vi "ClassPanel.vi"(8 "error in (no error)":errorcluster caption="entrée d'erreur (pas d'erreur)", 11 "SR530.lvclass":refnum<class "SR530.lvclass">) -> (0 "error out":errorcluster caption="sortie d'erreur", 3 "SR530.lvclass Out":refnum<class "SR530.lvclass">)   [LabVIEW 2019, in "SR530.lvclass"]
uses:
  SR530.lvclass
  C:/Programmes Labview/LabscanV1A/DevicesClass/BaseDevice/BaseDevice.lvclass
  <userlib>/SR530/Inputs.ctl
  <userlib>/SR530/ReadParam.ctl
  <userlib>/SR530/SetParam.ctl
  BaseDevice/ClassQueueMess.ctl
  BaseDevice/Accessor/GetClassEvent.vi
panel:
  in  "Read:":T1 items=["Channel 1", "X Output", "Channel 2", "Y Output", "X1", "X2", "X3", "X4", "X5", "X6", "Ch1 and Ch2", "X and Y", "X,Y,Ch1,Ch2"]
  in  "MainProgQ":refnum<queue>
  in  "MainProgQEvent":refnum<user-event>
  in  "Pre Time":u16(ring)=1 items=["1 ms"=1, "3 ms"=2, "10 ms"=3, "30 ms"=4, "100 ms"=5, "300 ms"=6, "1 s"=7, "3 s"=8, "10 s"=9, "30 s"=10, "100 s"=11]
  in  "Sensitivity":u16(ring)=1 items=["10 nV"=1, "20 nV"=2, "50 nV"=3, "100 nV"=4, "200 nV"=5, "500 nV"=6, "1 µV"=7, "2 µV"=8, "5 µV"=9, "10 µV"=10, "20 µV"=11, "50 µV"=12, "100µV"=13, "200 µV"=14, "500µV"=15, "1 mV"=16, "2 mV"=17, "5 mV"=18, "10 mV"=19, "20 mV"=20, "50 mV"=21, "100 mV"=22, "200mV"=23, "500 mV"=24]
  in  "Acq":bool
  out "Phase":dbl=1000.0 caption="Phase (°)" min=0.0 step=0.1 format="%#_5f"
  out "MAG":dbl=1000.0 caption="MAG (V)" min=0.0 step=0.1 format="%^#_6e"
  out "UNLCK":bool caption="SpexMov"
  out "X":dbl=1000.0 caption="X (V)" min=0.0 step=0.1 format="%^#_6e"
  in  "Stop":bool
  out "Init Program":bool
  out "OVLD":bool caption="SpexMov"
  in  "Update":bool caption="stopSpectro"
  out "Y":dbl=1000.0 caption="Y (V)" min=0.0 step=0.1 format="%^#_6e"
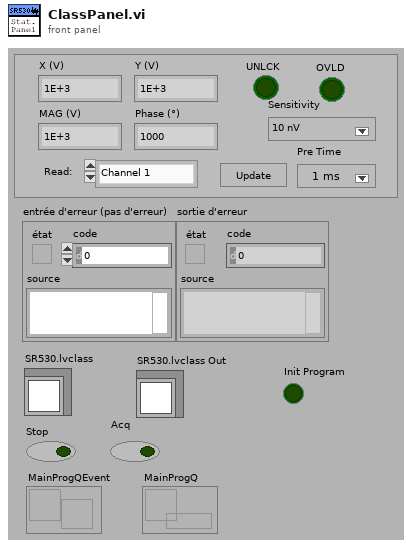
[diagram p1: front panel]
types:
  T1 = typedef "Inputs.ctl" = u16
  T2 = typedef "ReadParam.ctl" = enum16{"BandPass Filter", "Dynamic Reserve", "Expand", "Frequency", "Ref Trig", "Ch Settings", "Gain", "Notch Filter", "Time Constant", "All", "End"}
  T3 = typedef "SetParam.ctl" = enum16{"BandPass Filter", "Dynamic Reserve", "Expand", "Ref Trig", "Ch Settings", "Gain", "Notch Filter", "Pre Time Constant", "Post Time Constant"}
  T4 = cluster{"Channel":u16, "Outputs":dbl[], "Status Byte":bool[]}
  T5 = enum16{"Enable", "Disable", "DisAndGrayed", "ReinitToDefVal", "EnumElementsArr"}
  T6 = enum8{"Enabled", "Disabled", "Disabled and Grayed Out"}
  T7 = cluster{"BandFilter":bool, "LineFilter1x":bool, "LineFilter2x":bool, "Expand Ch1":bool, "Expand Ch2":bool, "Sensitivity":u16, "Pre Time":u16, "Post Time":u16, "Dynamic Res.":u16, "Reference Trigger":u16, "Channels Settings":u16, "Frequency":dbl}
  T8 = typedef "ClassQueueMess.ctl" = u16
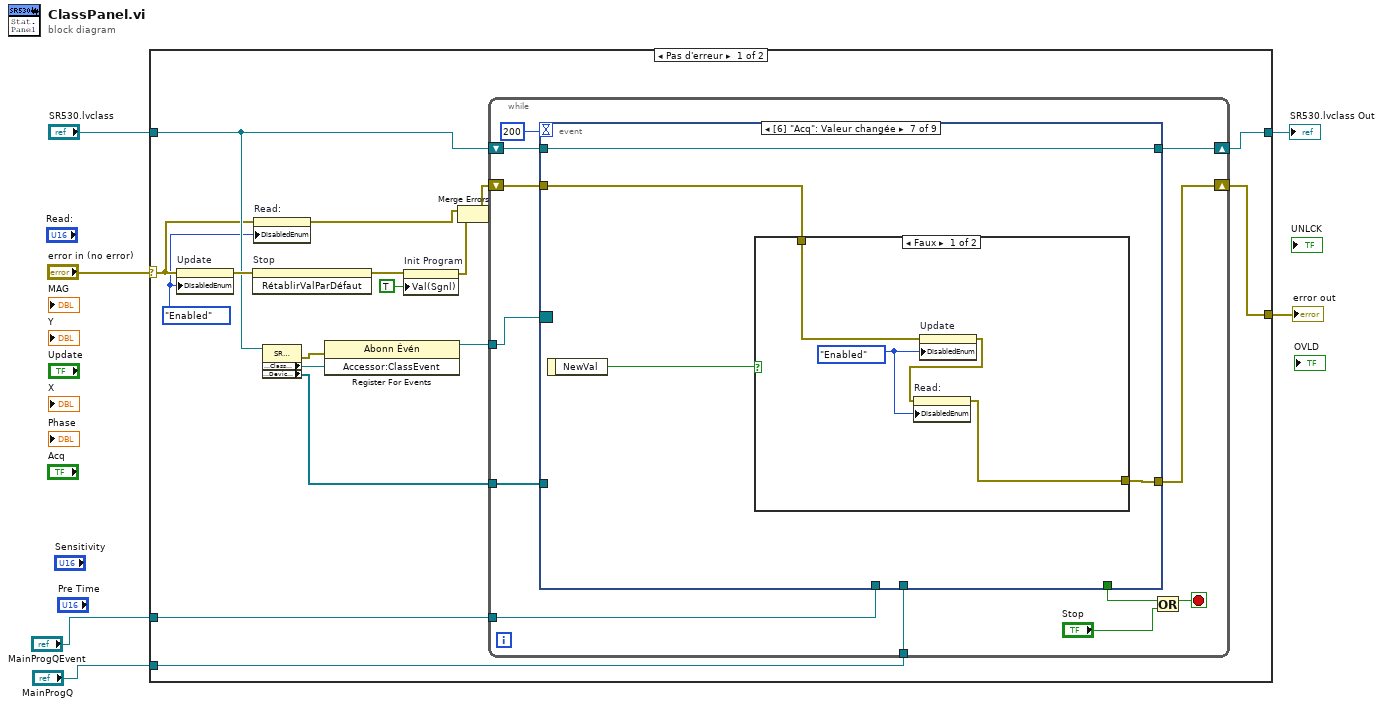
[diagram p0: block diagram]
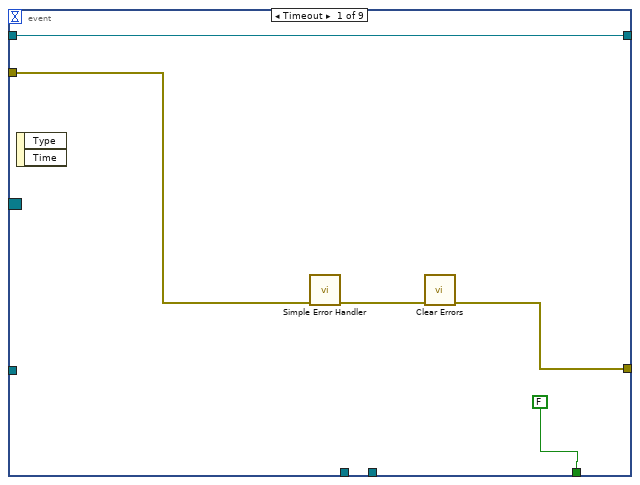
[diagram p2: hidden frame]
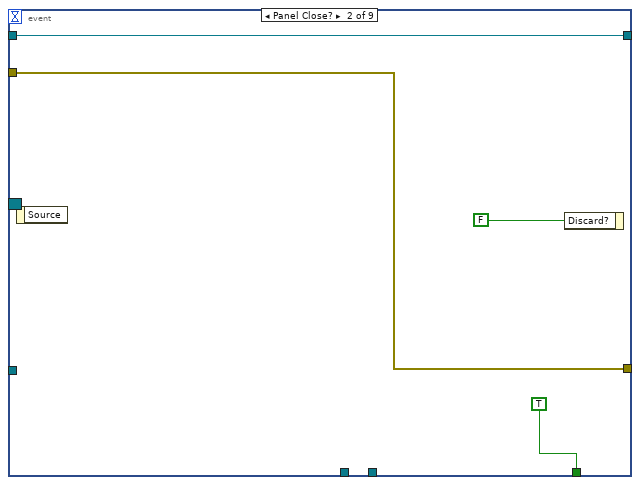
[diagram p3: hidden frame]
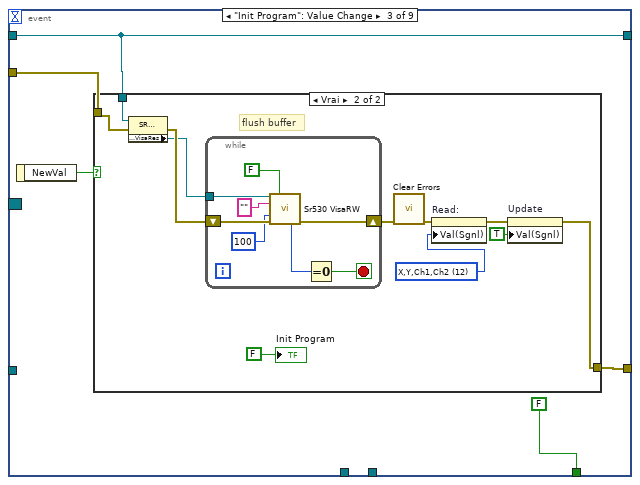
[diagram p4: hidden frame]
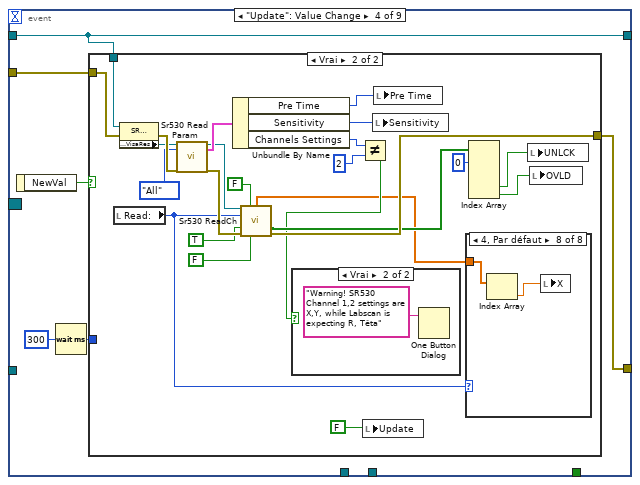
[diagram p6: hidden frame]
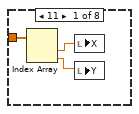
[diagram p8: hidden frame]
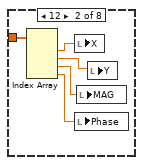
[diagram p9: hidden frame]
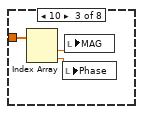
[diagram p10: hidden frame]
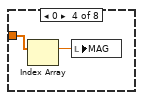
[diagram p11: hidden frame]
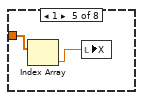
[diagram p12: hidden frame]
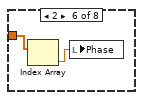
[diagram p13: hidden frame]
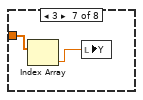
[diagram p14: hidden frame]
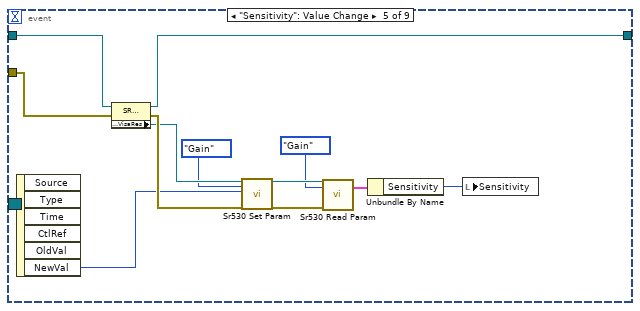
[diagram p16: hidden frame]
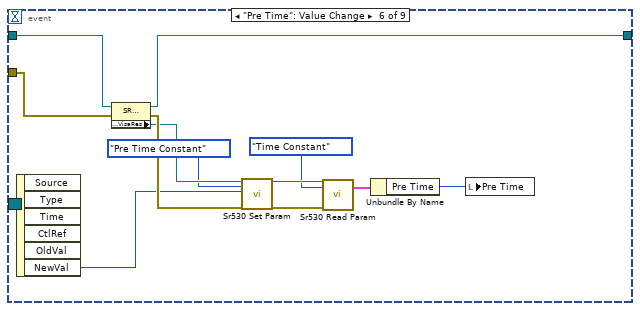
[diagram p17: hidden frame]
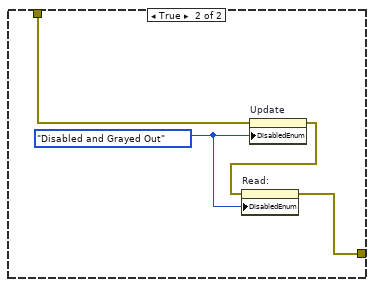
[diagram p18: hidden frame]
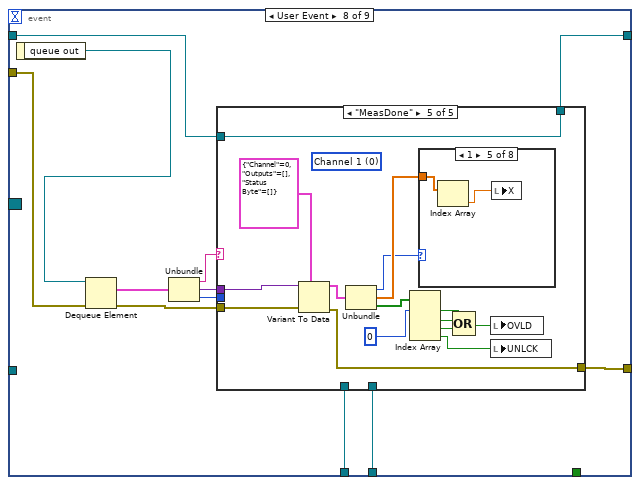
[diagram p19: hidden frame]
diagram:
  n1 = case shown="Pas d'erreur" "error in (no error)" {
    selector: "error in (no error)" -> [w10 w358]
    tunnel: [w14 w358] -> w5
    tunnel: "SR530.lvclass" -> [w15 w357]
    tunnel: [w22 w357] -> w3
    tunnel: "MainProgQEvent" -> [w13 _]
    tunnel: "MainProgQ" -> [w12 _]
    frame No Error {
      w7 = T6."Enabled" ("Désactivé")
      n2 = property on="Update" class="Bool (strict)"(error in=w10, "DisabledEnum"=w7) -> (error out=w18:errorcluster)  [unwired: 1 in, 1 out]
      n3 = invoke on="Stop" class="Bool (strict)" method="RétablirValParDéfaut"(error in=w18) -> (error out=w21:errorcluster)  [unwired: 2 in, 2 out]
      n4 = property on="Read:" class="MDér (strict)"(error in=w10, "DisabledEnum"=w7) -> (error out=w8:errorcluster)  [unwired: 1 in, 1 out]
      n5 = property class="SR530.lvclass"(reference=w15) -> (error out=w19:errorcluster, "Accessor:ClassEvent"=w20:refnum<user-event>, "Accessor:DeviceCtrl"=w11:refnum<vi>[])  [unwired: 1 in, 1 out]
      n6 = register-events(error in=w19, w20) -> (reference out=w17:refnum<event-registration>)  [unwired: 1 in, 1 out]
      n7 = property on="Init Program" class="Bool (strict)"(error in=w21, "Val(Sgnl)"=TRUE ("Valeur (Signalisation)")) -> (error out=w16:errorcluster)  [unwired: 1 in, 1 out]
      n8 = Merge Errors(w8, w16) -> (w9:errorcluster)
      n9 = while {
        shift-right: [w33] -> w14
        shift-left: w9 -> [w34]
        shift-right: [w30] -> w22
        shift-left: w15 -> [w32]
        tunnel: w17 -> [w27]
        tunnel: w13 -> [w26]
        tunnel: w12 -> [w25]
        tunnel: w11 -> [w24]
        stop <- w29 stop-if-true
        n10 = event shown="[6] \"Acq\": Valeur changée" {
          selector: w27 -> [_ _ _ _ _ _ _ _ _]
          dyn-events: _ -> [_ _ _ _ _ _ _ _ _]
          timeout: 200 -> [_ _ _ _ _ _ _ _ _]
          tunnel: w34 -> [w38 w42 w48 w70 w132 w144 w150 w168 w233]
          tunnel: [w36 w42 w47 w74 _ _ w148 w161 w234] -> w33
          tunnel: w32 -> [w39 w41 w45 w71 w133 w145 w147 w164 w242]
          tunnel: [FALSE TRUE FALSE _ _ _ _ _ _] -> w31
          tunnel: [w39 w41 w45 w71 w131 w143 w147 w163 w236] -> w30
          tunnel: w26 -> [_ _ _ _ _ _ _ w160 _]
          tunnel: w25 -> [_ _ _ _ _ _ _ w159 _]
          tunnel: w24 -> [_ _ _ _ _ _ _ _ w239]
          event Timeout {
            n11 = event-data() -> ()  [unwired: 1 in, 2 out]
            n12 = call <vilib>:"Simple Error Handler.vi"("error in (no error)"=w38) -> ("error out"=w37:errorcluster)  [unwired: 4 in, 4 out]
            n13 = call <vilib>:"Clear Errors.vi"("error in (no error)"=w37) -> ("error out"=w36:errorcluster)  [unwired: 5 in, 1 out]
          }
          event Panel Close? {
            n14 = event-data() -> ()  [unwired: 1 in, 1 out]
            n15 = event-data("Discard?"=FALSE ("Rejeter ?")) -> ()  [unwired: 1 in, 1 out]
          }
          event "Init Program": Value Change {
            n16 = event-data() -> ("NewVal"=w49:bool)  [unwired: 1 in]
            n17 = case shown="Vrai" w49 {
              tunnel: w48 -> [w50 w57]
              tunnel: [w50 w59] -> w47
              tunnel: w45 -> [_ w56]
              frame False {
              }
              frame True {
                w51 = T1 12 items=["Channel 1", "X Output", "Channel 2", "Y Output", "X1", "X2", "X3", "X4", "X5", "X6", "Ch1 and Ch2", "X and Y", "X,Y,Ch1,Ch2"] ("Read:")
                # "flush buffer"
                n18 = property class="SR530.lvclass"(reference=w56, error in=w57) -> (error out=w55:errorcluster, "Accessor:VisaRes"=w54:refnum<visa-resource-name>)  [unwired: 1 out]
                n19 = while {
                  tunnel: w54 -> [w68]
                  shift-right: [w64] -> w58
                  shift-left: w55 -> [w69]
                  stop <- w62 stop-if-true
                  n20 = call <userlib>:"Sr530 VisaRW.vi"("VISA Rsrc"=w68, "2Lecture?"=FALSE, "ChaineCom"="", "Nbcaract"=u32 100, "error in (no error)"=w69) -> ("Count out"=w63:u32, "error out"=w64:errorcluster)  [unwired: 5 in, 4 out]
                  n21 = Equal To 0?(x=w63) -> (x = 0?=w62:bool)
                }
                n22 = call <vilib>:"Clear Errors.vi"("error in (no error)"=w58) -> ("error out"=w52:errorcluster)  [unwired: 5 in, 1 out]
                n23 = property on="Read:" class="MDér (strict)"(error in=w52, "Val(Sgnl)"=w51) -> (error out=w53:errorcluster)  [unwired: 1 in, 1 out]
                n24 = property on="Update" class="Bool (strict)"(error in=w53, "Val(Sgnl)"=TRUE ("Valeur (Signalisation)")) -> (error out=w59:errorcluster)  [unwired: 1 in, 1 out]
                "Init Program" <- FALSE
              }
            }
          }
          event "Update": Value Change {
            n25 = event-data() -> ("NewVal"=w75:bool)  [unwired: 1 in]
            n26 = Wait (ms)(milliseconds to wait=u32 300 ("attente (ms)")) -> (millisecond timer value=w72:u32)
            n27 = case shown="Vrai" w75 {
              tunnel: w70 -> [w76 w93]
              tunnel: [w76 w87] -> w74
              tunnel: w72 -> [_ _]
              tunnel: w71 -> [_ w96]
              frame False {
              }
              frame True {
                n28 = local read "Read:"() -> (w78:T1)
                n29 = property class="SR530.lvclass"(reference=w96, error in=w93) -> (error out=w95:errorcluster, "Accessor:VisaRes"=w94:refnum<visa-resource-name>)  [unwired: 1 out]
                n30 = call <userlib>:"Sr530 Read Param.vi"("Ressource VISA"=w94, "Param"=ReadParam."All", "error in (no error)"=w95) -> ("Ressource VISA Out"=w91:refnum<visa-resource-name>, "LockInPar"=w100:T7, "error out"=w92:errorcluster)  [unwired: 13 in, 1 out]
                n31 = Unbundle By Name(w100) -> ("Pre Time"=w80:u16, "Sensitivity"=w99:u16, "Channels Settings"=w83:u16)
                n32 = call <userlib>:"Sr530 ReadCh.vi"("VISA Rsrc"=w91, "Autoscale"=FALSE, "Channel"=w78, "Check Status"=TRUE, "error in (no error)"=w92, "Ask Correction"=FALSE) -> ("Outputs"=w77:dbl[], "Status Byte"=w86:bool[], "error out"=w87:errorcluster)  [unwired: 2 in, 5 out]
                n33 = Not Equal?(x=w83, y=u16 2 ("Channels Settings")) -> (x != y?=w81:bool)
                n34 = case shown="Vrai" w81 {
                  frame False {
                  }
                  frame True {
                    n35 = One Button Dialog(message="Warning! SR530 Channel 1,2 settings are X,Y, while Labscan is expecting R, Têta") -> ()  [unwired: 1 in, 1 out]
                  }
                }
                n36 = local write "Update"(FALSE) -> ()
                n37 = local write "Sensitivity"(w99) -> ()
                n38 = local write "Pre Time"(w80) -> ()
                n39 = case shown="4, Par défaut" w78 {
                  tunnel: w77 -> [w101 w106 w109 w113 w115 w117 w119 w120]
                  frame 11 {
                    n40 = Index Array(array=w101) -> (element #1=w103:dbl, element #2=w102:dbl)  [unwired: 2 in]
                    n41 = local write "X"(w103) -> ()
                    n42 = local write "Y"(w102) -> ()
                  }
                  frame 12 {
                    n43 = Index Array(array=w106) -> (element #1=w108:dbl, element #2=w107:dbl, element #3=w105:dbl, element #4=w104:dbl)  [unwired: 4 in]
                    n44 = local write "X"(w108) -> ()
                    n45 = local write "Phase"(w104) -> ()
                    n46 = local write "MAG"(w105) -> ()
                    n47 = local write "Y"(w107) -> ()
                  }
                  frame 10 {
                    n48 = Index Array(array=w109) -> (element #1=w111:dbl, element #2=w110:dbl)  [unwired: 2 in]
                    n49 = local write "Phase"(w110) -> ()
                    n50 = local write "MAG"(w111) -> ()
                  }
                  frame 0 {
                    n51 = Index Array(array=w113) -> (element=w112:dbl)  [unwired: 1 in]
                    n52 = local write "MAG"(w112) -> ()
                  }
                  frame 1 {
                    n53 = Index Array(array=w115) -> (element=w114:dbl)  [unwired: 1 in]
                    n54 = local write "X"(w114) -> ()
                  }
                  frame 2 {
                    n55 = Index Array(array=w117) -> (element=w116:dbl)  [unwired: 1 in]
                    n56 = local write "Phase"(w116) -> ()
                  }
                  frame 3 {
                    n57 = Index Array(array=w119) -> (element=w118:dbl)  [unwired: 1 in]
                    n58 = local write "Y"(w118) -> ()
                  }
                  frame 4, Default {
                    n59 = Index Array(array=w120) -> (element=w121:dbl)  [unwired: 1 in]
                    n60 = local write "X"(w121) -> ()
                  }
                }
                n61 = Index Array(array=w86, index #1=0 ("indice")) -> (element #4=w84:bool, element #5=w85:bool)  [unwired: 4 in, 3 out]
                n62 = local write "UNLCK"(w84) -> ()
                n63 = local write "OVLD"(w85) -> ()
              }
            }
          }
          event "Sensitivity": Value Change {
            n64 = event-data() -> ("NewVal"=w127:u16)  [unwired: 1 in, 5 out]
            n65 = property class="SR530.lvclass"(reference=w133, error in=w132) -> (reference out=w131:refnum<class "SR530.lvclass">, error out=w130:errorcluster, "Accessor:VisaRes"=w129:refnum<visa-resource-name>)
            n66 = call <userlib>:"Sr530 Set Param.vi"("Ressource VISA"=w129, "Param"=SetParam."Gain", "Sensitivity"=w127, "error in (no error)"=w130) -> ("Ressource VISA Out"=w134:refnum<visa-resource-name>, "error out"=w126:errorcluster)  [unwired: 14 in]
            n67 = call <userlib>:"Sr530 Read Param.vi"("Ressource VISA"=w134, "Param"=ReadParam."Gain", "error in (no error)"=w126) -> ("LockInPar"=w124:T7)  [unwired: 13 in, 3 out]
            n68 = Unbundle By Name(w124) -> ("Sensitivity"=w123:u16)
            n69 = local write "Sensitivity"(w123) -> ()
          }
          event "Pre Time": Value Change {
            n70 = event-data() -> ("NewVal"=w139:u16)  [unwired: 1 in, 5 out]
            n71 = property class="SR530.lvclass"(reference=w145, error in=w144) -> (reference out=w143:refnum<class "SR530.lvclass">, error out=w142:errorcluster, "Accessor:VisaRes"=w141:refnum<visa-resource-name>)
            n72 = call <userlib>:"Sr530 Set Param.vi"("Ressource VISA"=w141, "Param"=SetParam."Pre Time Constant", "Sensitivity"=w139, "error in (no error)"=w142) -> ("Ressource VISA Out"=w146:refnum<visa-resource-name>, "error out"=w138:errorcluster)  [unwired: 14 in]
            n73 = call <userlib>:"Sr530 Read Param.vi"("Ressource VISA"=w146, "Param"=ReadParam."Time Constant", "error in (no error)"=w138) -> ("LockInPar"=w136:T7)  [unwired: 13 in, 3 out]
            n74 = Unbundle By Name(w136) -> ("Pre Time"=w135:u16)
            n75 = local write "Pre Time"(w135) -> ()
          }
          event "Acq": Value Change {
            n76 = event-data() -> ("NewVal"=w149:bool)  [unwired: 1 in]
            n77 = case shown="Faux" w149 {
              tunnel: w150 -> [w154 w158]
              tunnel: [w151 w155] -> w148
              frame False {
                w152 = T6."Enabled" ("Désactivé")
                n78 = property on="Update" class="Bool (strict)"(error in=w154, "DisabledEnum"=w152) -> (error out=w153:errorcluster)  [unwired: 1 in, 1 out]
                n79 = property on="Read:" class="MDér (strict)"(error in=w153, "DisabledEnum"=w152) -> (error out=w151:errorcluster)  [unwired: 1 in, 1 out]
              }
              frame True {
                w157 = T6."Disabled and Grayed Out" ("Désactivé")
                n80 = property on="Update" class="Bool (strict)"(error in=w158, "DisabledEnum"=w157) -> (error out=w156:errorcluster)  [unwired: 1 in, 1 out]
                n81 = property on="Read:" class="MDér (strict)"(error in=w156, "DisabledEnum"=w157) -> (error out=w155:errorcluster)  [unwired: 1 in, 1 out]
              }
            }
          }
          event User Event {
            n82 = event-data() -> ("queue out"=w169:refnum<queue>)  [unwired: 1 in]
            n83 = Dequeue Element(queue=w169, error in (no error)=w168) -> (element=w170:cluster{"Message":string, "Data":variant, i32}, error out=w162:errorcluster)  [unwired: 1 in, 2 out]
            n84 = Unbundle(w170) -> ("Message"=w167:string, "Data"=w166:variant, w165:i32)
            n85 = case shown="\"MeasDone\"" w167 {
              tunnel: w166 -> [_ _ w180 _ w205]
              tunnel: w165 -> [_ _ _ _ _]
              tunnel: w164 -> [w172 w177 w182 w187 w206]
              tunnel: [w172 w177 w181 w187 w206] -> w163
              tunnel: w162 -> [w171 w174 w179 w186 w204]
              tunnel: [w171 w173 w178 w185 w203] -> w161
              tunnel: w160 -> [_ _ _ w184 _]
              tunnel: w159 -> [_ _ _ w183 _]
              frame Default {
              }
              frame "ShowDiag" {
                n86 = control-ref of="This VI"() -> (w175:refnum<vi>)
                n87 = call <userlib>:"AnimExecGen.vi"("ErrorIn(No Error)"=w174, "Animer l'exécution ?"=TRUE, "ViRef"=w175) -> ("sortie d'erreur"=w173:errorcluster)  [unwired: 8 in]
              }
              frame "UpdateClassData" {
                n88 = Variant To Data(error in=w179, type=w182, Variant=w180) -> (data=w181:refnum<class "SR530.lvclass">, error out=w178:errorcluster)
              }
              frame "UpdateMainClass" {
                n89 = Bundle By Name(cluster=cluster{"Message":string, "Data":variant, i32} {"Message"="", "Data"=variant, 0} ("élément"), "Data"=w187) -> (w188:cluster{"Message":string, "Data":variant, i32})
                n90 = Enqueue Element(queue=w183, element=w188, error in (no error)=w186) -> (queue out=w191:refnum<queue>, error out=w190:errorcluster)  [unwired: 1 in, 1 out]
                n91 = Generate User Event(user event=w184, event data cluster=w191, error in=w190) -> (error out=w185:errorcluster)  [unwired: 1 in, 1 out]
              }
              frame "MeasDone" {
                (unwired) T1 0 items=["Channel 1", "X Output", "Channel 2", "Y Output", "X1", "X2", "X3", "X4", "X5", "X6", "Ch1 and Ch2", "X and Y", "X,Y,Ch1,Ch2"] ("Channel")
                n92 = Variant To Data(error in=w204, type=T4 {"Channel"=0, "Outputs"=[], "Status Byte"=[]} ("cluster"), Variant=w205) -> (data=w202:T4, error out=w203:errorcluster)
                n93 = Unbundle(w202) -> ("Channel"=w193:u16, "Outputs"=w194:dbl[], "Status Byte"=w192:bool[])
                n94 = Index Array(array=w192, index #1=0 ("indice")) -> (element #1=w200:bool, element #2=w199:bool, element #3=w198:bool, element #4=w201:bool)  [unwired: 3 in]
                n95 = case shown="1" w193 {
                  tunnel: w194 -> [w207 w212 w215 w219 w221 w223 w225 w226]
                  frame 11 {
                    n96 = Index Array(array=w207) -> (element #1=w209:dbl, element #2=w208:dbl)  [unwired: 2 in]
                    n97 = local write "X"(w209) -> ()
                    n98 = local write "Y"(w208) -> ()
                  }
                  frame 12 {
                    n99 = Index Array(array=w212) -> (element #1=w214:dbl, element #2=w213:dbl, element #3=w211:dbl, element #4=w210:dbl)  [unwired: 4 in]
                    n100 = local write "X"(w214) -> ()
                    n101 = local write "Phase"(w210) -> ()
                    n102 = local write "MAG"(w211) -> ()
                    n103 = local write "Y"(w213) -> ()
                  }
                  frame 10 {
                    n104 = Index Array(array=w215) -> (element #1=w217:dbl, element #2=w216:dbl)  [unwired: 2 in]
                    n105 = local write "Phase"(w216) -> ()
                    n106 = local write "MAG"(w217) -> ()
                  }
                  frame 0 {
                    n107 = Index Array(array=w219) -> (element=w218:dbl)  [unwired: 1 in]
                    n108 = local write "MAG"(w218) -> ()
                  }
                  frame 1 {
                    n109 = Index Array(array=w221) -> (element=w220:dbl)  [unwired: 1 in]
                    n110 = local write "X"(w220) -> ()
                  }
                  frame 2 {
                    n111 = Index Array(array=w223) -> (element=w222:dbl)  [unwired: 1 in]
                    n112 = local write "Phase"(w222) -> ()
                  }
                  frame 3 {
                    n113 = Index Array(array=w225) -> (element=w224:dbl)  [unwired: 1 in]
                    n114 = local write "Y"(w224) -> ()
                  }
                  frame 4, Default {
                    n115 = Index Array(array=w226) -> (element=w227:dbl)  [unwired: 1 in]
                    n116 = local write "X"(w227) -> ()
                  }
                }
                n117 = Compound Arithmetic op=OR(w200, w199, w198) -> (w197:bool)
                n118 = local write "OVLD"(w197) -> ()
                n119 = local write "UNLCK"(w201) -> ()
              }
            }
          }
          event Value Change {
            w238 = T8 1 items=["UpdateClassData", "UpdateMainClass"] ("Menu déroulant")
            n120 = event-data() -> ("NewVal"=w241:T1)  [unwired: 1 in]
            n121 = Index Array(array=w239) -> (element=w229:refnum<vi>)  [unwired: 1 in]
            n122 = case shown="0" w241 {
              selector: w241 -> [_ _ _ _ w319 _ _ _]
              tunnel: [string[] ["Mag(V)"] string[] ["X(V)"] string[] ["Phase(°)"] string[] ["Y(V)"] w306 string[] ["Mag(V)", "Phase(°)"] string[] ["X(V)", "Y(V)"] string[] ["X(V)", "Y(V)", "Mag(V)", "Phase(°)"]] -> w240
              tunnel: w239 -> [w255 w263 w277 w291 w311 w323 w337 w355]
              tunnel: w233 -> [w256 w262 w276 w290 w316 w322 w336 w351]
              tunnel: [w247 w261 w275 w289 w307 w321 w335 w349] -> w232
              tunnel: [_ _ _ _ w305 _ _ _] -> w231
              tunnel: [_ _ _ _ TRUE _ _ _] -> w230
              tunnel: w229 -> [_ _ _ _ w303 _ _ _]
              frame 0 {
                n123 = Delete From Array(array=w255, length=4 ("longueur"), index=0 ("indice")) -> (deleted portion=w254:refnum<vi>[])  [unwired: 1 out]
                n124 = Delete From Array(array=w254, length=1 ("longueur"), index=2 ("indice")) -> (deleted portion=w250:refnum<vi>[], array with subset deleted=w251:refnum<vi>[])
                n125 = call <userlib>:"SetCtrlPropGen.vi"("Error in"=w256, "Énum"=T5."DisAndGrayed", "Controls"=w251) -> ("Error out"=w249:errorcluster)  [unwired: 3 in, 1 out]
                n126 = call <userlib>:"SetCtrlPropGen.vi"("Error in"=w249, "Énum"=T5."Enable", "Controls"=w250) -> ("Error out"=w247:errorcluster)  [unwired: 3 in, 1 out]
              }
              frame 1 {
                n127 = Delete From Array(array=w263, length=4 ("longueur"), index=0 ("indice")) -> (deleted portion=w270:refnum<vi>[])  [unwired: 1 out]
                n128 = Delete From Array(array=w270, length=1 ("longueur"), index=0 ("indice")) -> (deleted portion=w266:refnum<vi>[], array with subset deleted=w267:refnum<vi>[])
                n129 = call <userlib>:"SetCtrlPropGen.vi"("Error in"=w262, "Énum"=T5."DisAndGrayed", "Controls"=w267) -> ("Error out"=w265:errorcluster)  [unwired: 3 in, 1 out]
                n130 = call <userlib>:"SetCtrlPropGen.vi"("Error in"=w265, "Énum"=T5."Enable", "Controls"=w266) -> ("Error out"=w261:errorcluster)  [unwired: 3 in, 1 out]
              }
              frame 2 {
                n131 = Delete From Array(array=w277, length=4 ("longueur"), index=0 ("indice")) -> (deleted portion=w284:refnum<vi>[])  [unwired: 1 out]
                n132 = Delete From Array(array=w284, length=1 ("longueur"), index=3 ("indice")) -> (deleted portion=w280:refnum<vi>[], array with subset deleted=w281:refnum<vi>[])
                n133 = call <userlib>:"SetCtrlPropGen.vi"("Error in"=w276, "Énum"=T5."DisAndGrayed", "Controls"=w281) -> ("Error out"=w279:errorcluster)  [unwired: 3 in, 1 out]
                n134 = call <userlib>:"SetCtrlPropGen.vi"("Error in"=w279, "Énum"=T5."Enable", "Controls"=w280) -> ("Error out"=w275:errorcluster)  [unwired: 3 in, 1 out]
              }
              frame 3 {
                n135 = Delete From Array(array=w291, length=4 ("longueur"), index=0 ("indice")) -> (deleted portion=w298:refnum<vi>[])  [unwired: 1 out]
                n136 = Delete From Array(array=w298, length=1 ("longueur"), index=1 ("indice")) -> (deleted portion=w294:refnum<vi>[], array with subset deleted=w295:refnum<vi>[])
                n137 = call <userlib>:"SetCtrlPropGen.vi"("Error in"=w290, "Énum"=T5."DisAndGrayed", "Controls"=w295) -> ("Error out"=w293:errorcluster)  [unwired: 3 in, 1 out]
                n138 = call <userlib>:"SetCtrlPropGen.vi"("Error in"=w293, "Énum"=T5."Enable", "Controls"=w294) -> ("Error out"=w289:errorcluster)  [unwired: 3 in, 1 out]
              }
              frame 4..9 {
                n139 = property on="Read:" class="MDér (strict)"(error in=w316) -> (error out=w315:errorcluster, "Strings []"=w320:string[])  [unwired: 1 in, 1 out]
                n140 = Index Array(array=w320, index=w319) -> (element=w318:string)
                n141 = Delete From Array(array=w311, length=3 ("longueur"), index=1 ("indice")) -> (deleted portion=w310:refnum<vi>[])  [unwired: 1 out]
                n142 = call <userlib>:"SetCtrlPropGenSgl.vi"("Error in"=w315, "Énum"=T5."Enable", "Controls"=w303) -> ("Error out"=w308:errorcluster)  [unwired: 3 in, 1 out]
                n143 = Concatenate Strings(w318, "(V)" ("chaîne")) -> (w305:string)
                n144 = Build Array(w305) -> (w306:string[])
                n145 = call <userlib>:"SetCtrlPropGen.vi"("Error in"=w308, "Énum"=T5."DisAndGrayed", "Controls"=w310) -> ("Error out"=w307:errorcluster)  [unwired: 3 in, 1 out]
              }
              frame 10 {
                n146 = Delete From Array(array=w323, length=4 ("longueur"), index=0 ("indice")) -> (deleted portion=w330:refnum<vi>[])  [unwired: 1 out]
                n147 = Delete From Array(array=w330, length=2 ("longueur"), index=2 ("indice")) -> (deleted portion=w326:refnum<vi>[], array with subset deleted=w327:refnum<vi>[])
                n148 = call <userlib>:"SetCtrlPropGen.vi"("Error in"=w322, "Énum"=T5."DisAndGrayed", "Controls"=w327) -> ("Error out"=w325:errorcluster)  [unwired: 3 in, 1 out]
                n149 = call <userlib>:"SetCtrlPropGen.vi"("Error in"=w325, "Énum"=T5."Enable", "Controls"=w326) -> ("Error out"=w321:errorcluster)  [unwired: 3 in, 1 out]
              }
              frame 11 {
                n150 = Delete From Array(array=w337, length=4 ("longueur"), index=0 ("indice")) -> (deleted portion=w344:refnum<vi>[])  [unwired: 1 out]
                n151 = Delete From Array(array=w344, length=2 ("longueur"), index=0 ("indice")) -> (deleted portion=w340:refnum<vi>[], array with subset deleted=w341:refnum<vi>[])
                n152 = call <userlib>:"SetCtrlPropGen.vi"("Error in"=w336, "Énum"=T5."DisAndGrayed", "Controls"=w341) -> ("Error out"=w339:errorcluster)  [unwired: 3 in, 1 out]
                n153 = call <userlib>:"SetCtrlPropGen.vi"("Error in"=w339, "Énum"=T5."Enable", "Controls"=w340) -> ("Error out"=w335:errorcluster)  [unwired: 3 in, 1 out]
              }
              frame 12, Default {
                n154 = Delete From Array(array=w355, length=4 ("longueur"), index=0 ("indice")) -> (deleted portion=w352:refnum<vi>[])  [unwired: 1 out]
                n155 = call <userlib>:"SetCtrlPropGen.vi"("Error in"=w351, "Énum"=T5."Enable", "Controls"=w352) -> ("Error out"=w349:errorcluster)  [unwired: 3 in, 1 out]
              }
            }
            n156 = property class="SR530.lvclass"(reference=w242, error in=w232, "Accessor:DataNames"=w240, "Accessor:DatDisplayNm"=string[] [] ("DatDisplayNm")) -> (reference out=w237:refnum<class "SR530.lvclass">, error out=w235:errorcluster)
            n157 = case shown="Vrai" w230 {
              tunnel: w231 -> [_ w246]
              tunnel: w229 -> [w243 w245]
              frame False {
                n158 = property class="Cmde"(reference=w243, "Caption.Text"="X (V)" ("chaîne")) -> ()  [unwired: 1 in, 2 out]
              }
              frame True {
                n159 = property class="Cmde"(reference=w245, "Caption.Text"=w246) -> ()  [unwired: 1 in, 2 out]
              }
            }
            n160 = call-dynamic "SetClassQueueMessage.vi"("ErrorIn(No Error)"=w235, "Menu déroulant"=w238, "DefaultDev.lvclass"=w237) -> ("sortie d'erreur"=w234:errorcluster, "DefaultDev.lvclass Out"=w236:refnum<class "SR530.lvclass">)  [unwired: 7 in]
          }
        }
        n161 = Or(x=w31, y="Stop") -> (x .or. y?=w29:bool)
      }
    }
    frame Error {
    }
  }
  "error out" <- w5
  "SR530.lvclass Out" <- w3
